vi "DVW_Read Waveform.vi"(3 "DVW":T2) -> (1 "Raw Data Waveform Out":T1)   [LabVIEW 2020]
uses:
  TypeDefs_Utility/Ref_DVR_Buffer.ctl
  Universal Controls/Waveform_Data.ctl
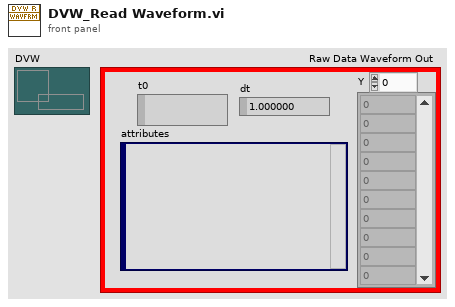
[diagram p1: front panel]
types:
  T1 = typedef "Waveform_Data.ctl" = waveform(dbl)
  T2 = typedef "Ref_DVR_Buffer.ctl" = refnum<data-value>
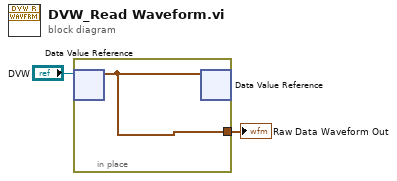
[diagram p0: block diagram]
diagram:
  n1 = in-place {
    in-place-border: [w3] -> w1
    n2 = in-place-dvr #1("DVW") -> (w3:T1)  [unwired: 1 out]
    n3 = in-place-dvr #1(w3) -> ()  [unwired: 2 out]
  }
  "Raw Data Waveform Out" <- w1
